vi "command-processor-old.vi"(8 "error in":errorcluster, 10 "Message Data Varient":variant, 11 "Queue in":refnum<queue>) -> (0 "error out":errorcluster, 1 "delta":dbl, 2 "executing command":string, 3 "output cluster":T1)   [LabVIEW 2017]
uses:
  Message Queue/Message Queue.lvlib
  Message Queue/Enqueue Message (Single).vi
  event-message-data.ctl
  Message Queue/Message Cluster.ctl
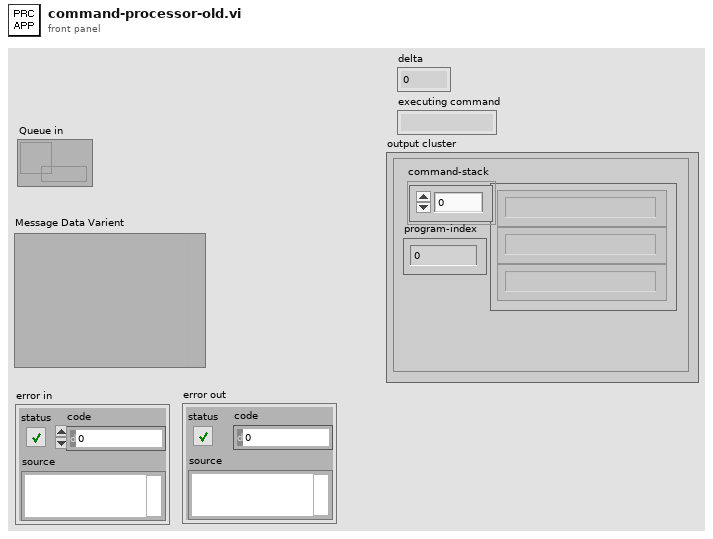
[diagram p1: front panel]
types:
  T1 = typedef "event-message-data.ctl" = cluster{"command-stack":string[], "program-index":i64}
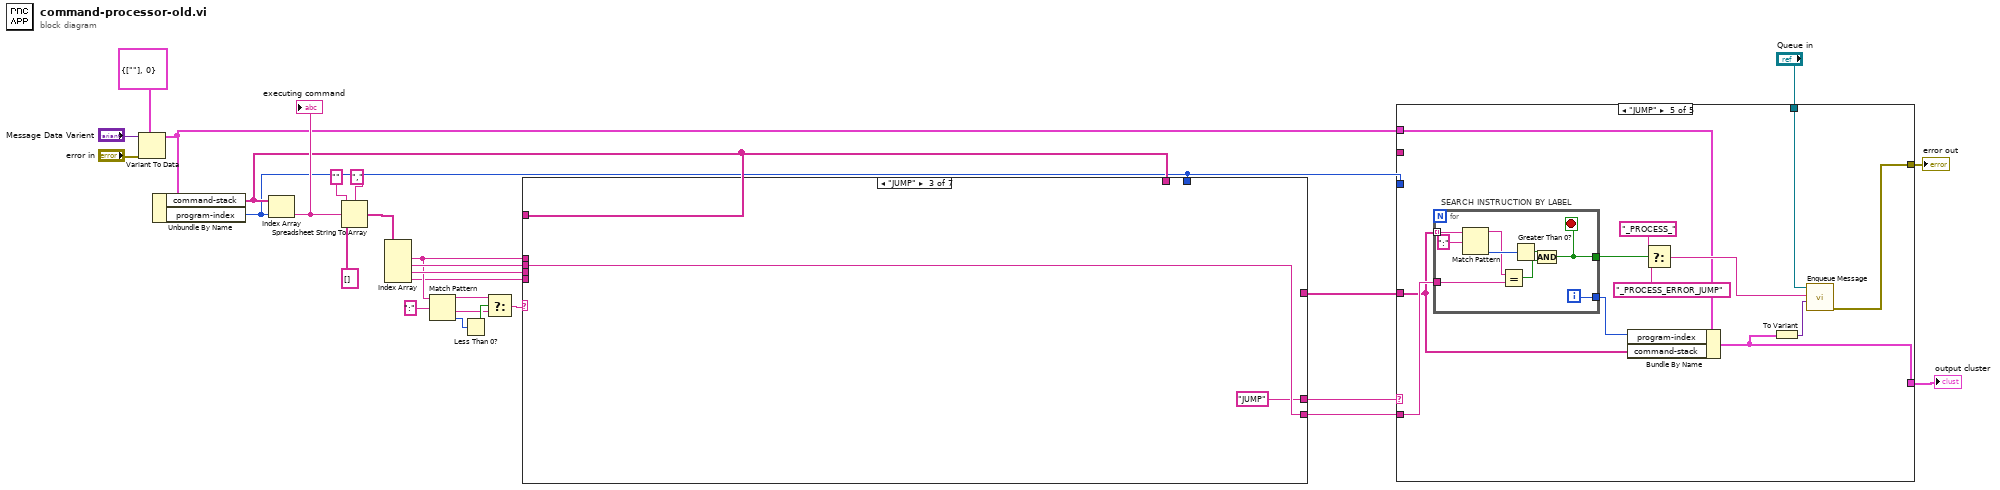
[diagram p0: block diagram]
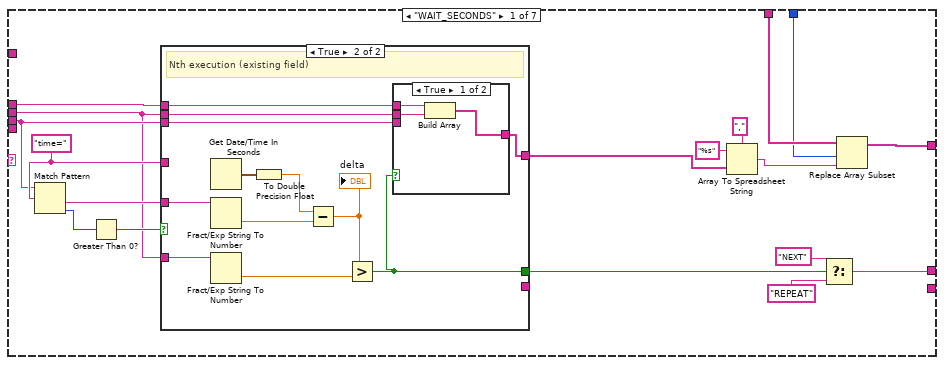
[diagram p2: hidden frame]
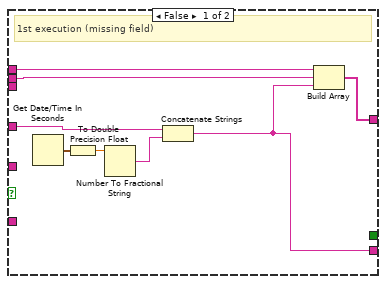
[diagram p3: hidden frame]
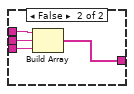
[diagram p4: hidden frame]
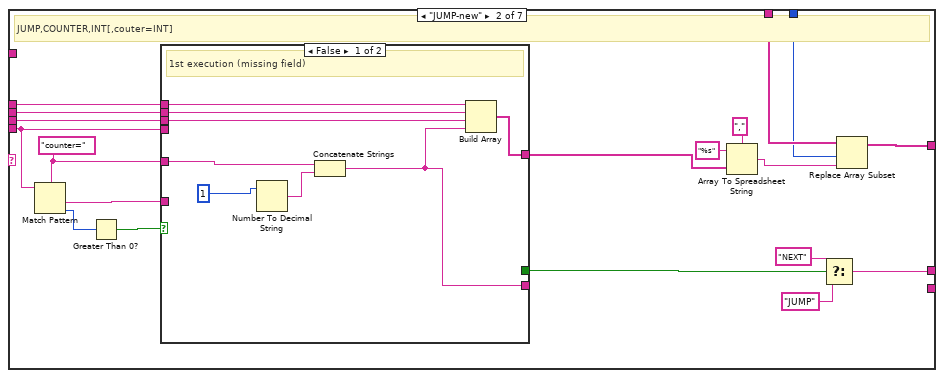
[diagram p5: hidden frame]
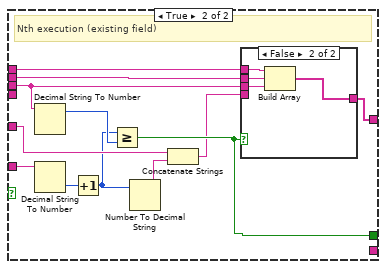
[diagram p6: hidden frame]
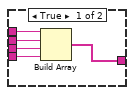
[diagram p7: hidden frame]
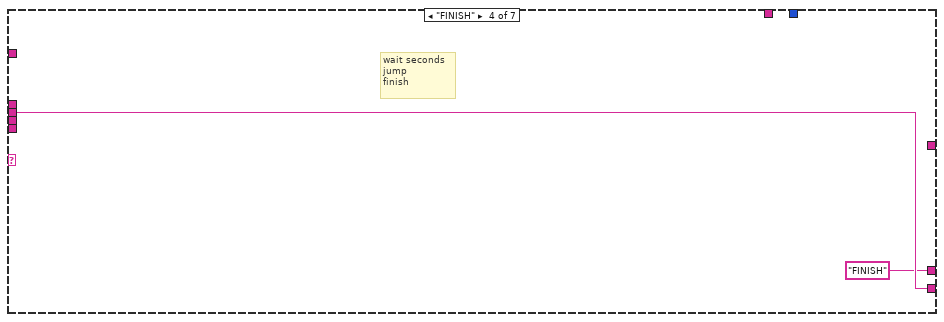
[diagram p8: hidden frame]
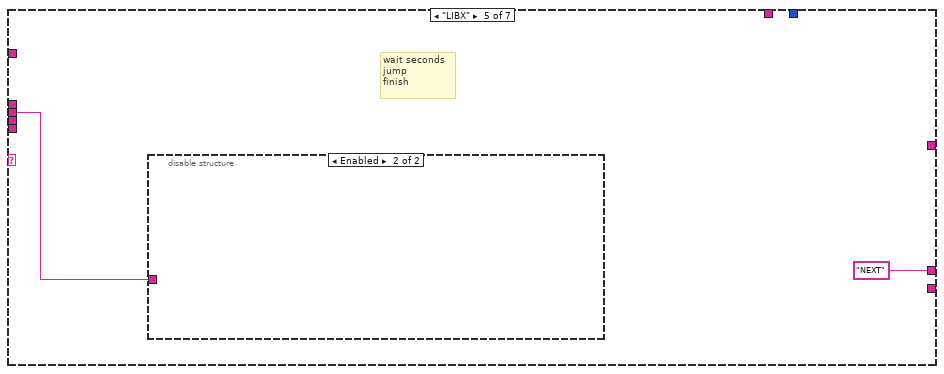
[diagram p9: hidden frame]
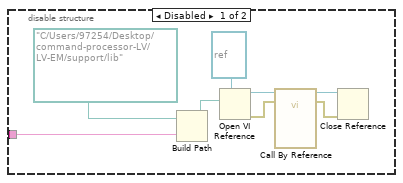
[diagram p10: hidden frame]
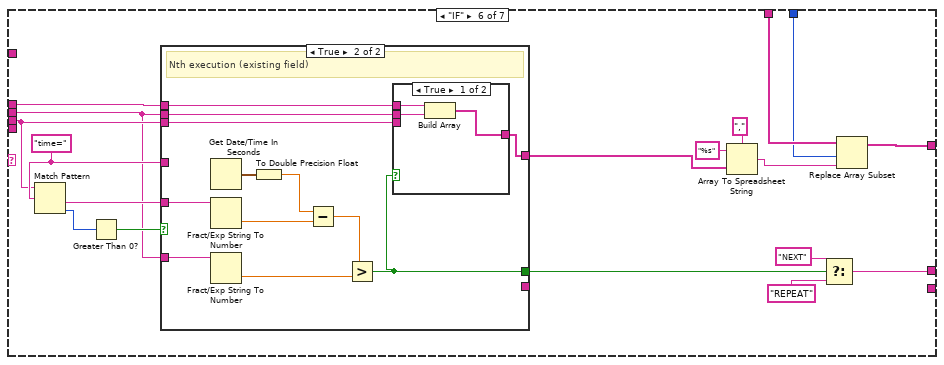
[diagram p11: hidden frame]
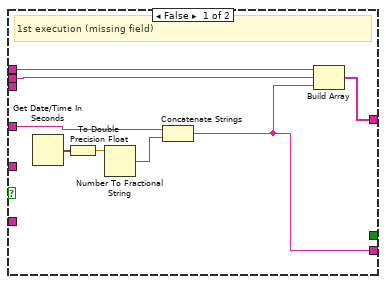
[diagram p12: hidden frame]
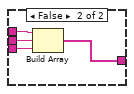
[diagram p13: hidden frame]
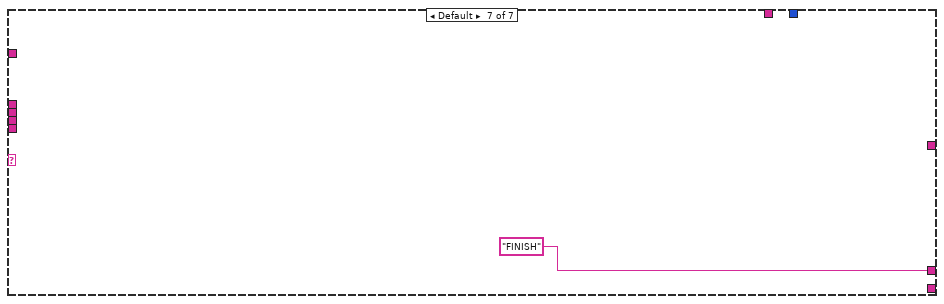
[diagram p14: hidden frame]
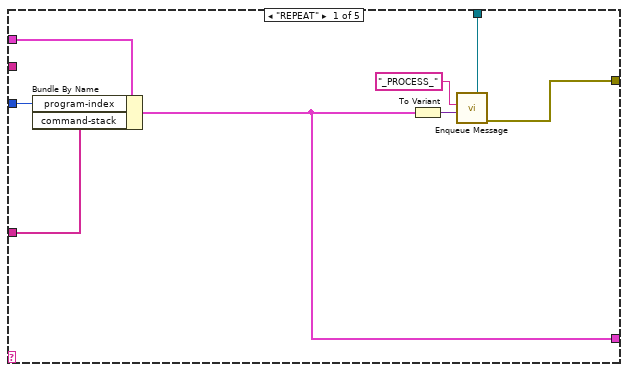
[diagram p15: hidden frame]
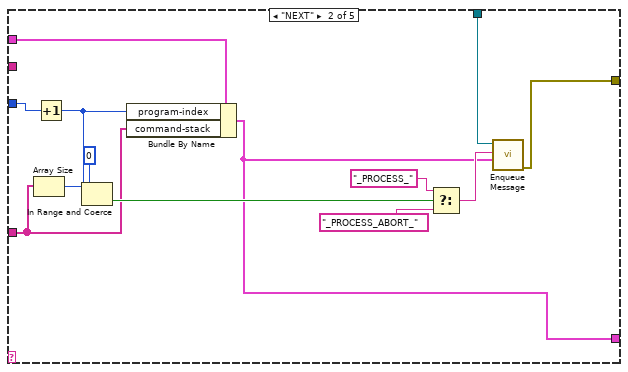
[diagram p16: hidden frame]
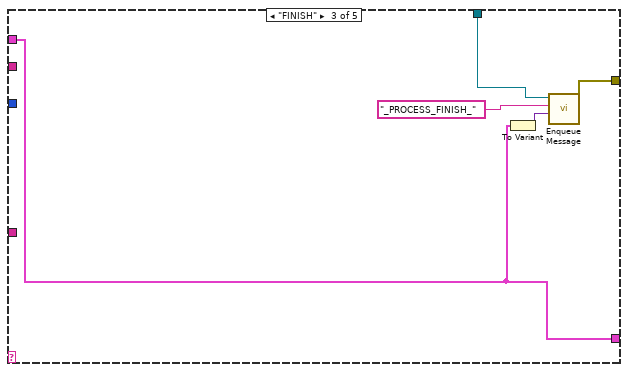
[diagram p17: hidden frame]
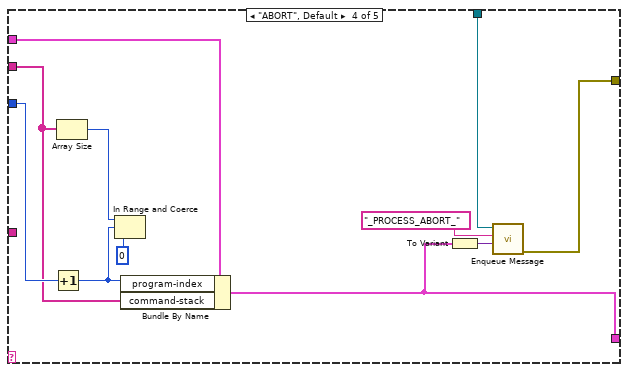
[diagram p18: hidden frame]
diagram:
  n1 = Variant To Data(error in="error in", type=T1 {"command-stack"=[""], "program-index"=0} ("process-unit"), Variant="Message Data Varient") -> (data=w5:T1)  [unwired: 1 out]
  n2 = Unbundle By Name(w5) -> ("command-stack"=w4:string[], "program-index"=w3:i64)
  n3 = Index Array(array=w4, index=w3) -> (element=w17:string)
  "executing command" <- w17
  n4 = Spreadsheet String To Array(delimiter (Tab)=",", format string="", spreadsheet string=w17, array type (2D Dbl)=string[] []) -> (array=w18:string[])
  n5 = Index Array(array=w18) -> (element #1=w6:string, element #2=w16:string, element #3=w15:string, element #4=w1:string)  [unwired: 4 in]
  n6 = Match Pattern(string=w6, regular expression=":") -> (before substring=w11:string, after substring=w10:string, offset past match=w13:i32)  [unwired: 1 in, 1 out]
  n7 = Less Than 0?(x=w13) -> (x < 0?=w12:bool)
  n8 = Select(t=w11, s=w12, f=w10) -> (s? t:f=w9:string)
  n9 = case shown="\"JUMP\"" w9 {
    tunnel: [w41 w87 "JUMP" ("format string") "FINISH" ("format string") "NEXT" ("format string") w148 "FINISH" ("format string")] -> w26
    tunnel: w16 -> [w33 w80 w122 w124 w125 w140 _]
    tunnel: w15 -> [w40 w86 _ _ _ w147 _]
    tunnel: [_ _ w122 w124 _ _ _] -> w8
    tunnel: w4 -> [_ _ _ _ _ _ _]
    tunnel: w6 -> [w34 w81 _ _ _ w141 _]
    tunnel: w4 -> [w31 w78 _ _ _ w138 _]
    tunnel: w3 -> [w29 w76 _ _ _ w136 _]
    tunnel: [w28 w75 _ _ _ w135 _] -> w2
    tunnel: w1 -> [_ w73 _ _ _ _ _]
    frame "WAIT_SECONDS" {
      w42 = "time=" ("regular expression")
      n10 = Match Pattern(string=w40, regular expression=w42) -> (after substring=w43:string, offset past match=w45:i32)  [unwired: 1 in, 2 out]
      n11 = Greater Than 0?(x=w45) -> (x > 0?=w44:bool)
      n12 = case shown="True" w44 {
        tunnel: [w47 _] -> _
        tunnel: w43 -> [_ w55]
        tunnel: w33 -> [_ w61]
        tunnel: w40 -> [_ w54]
        tunnel: w42 -> [w50 _]
        tunnel: [_ w59] -> w35
        tunnel: w34 -> [w49 w57]
        tunnel: w33 -> [w48 w56]
        tunnel: [w46 w58] -> w32
        frame False {
          # "1st execution (missing field)"
          n13 = Get Date/Time In Seconds() -> (seconds since 1Jan1904=w53:timestamp)
          n14 = To Double Precision Float(number=w53) -> (double precision float=w52:dbl)
          n15 = Number To Fractional String(number=w52) -> (F-format string=w51:string)  [unwired: 3 in]
          n16 = Concatenate Strings(w50, w51) -> (w47:string)
          n17 = Build Array(w49, w48, w47) -> (w46:string[])
        }
        frame True {
          # "Nth execution (existing field)"
          n18 = Get Date/Time In Seconds() -> (seconds since 1Jan1904=w65:timestamp)
          n19 = Fract/Exp String To Number(string=w55) -> (number=w63:dbl)  [unwired: 3 in, 1 out]
          n20 = Fract/Exp String To Number(string=w61) -> (number=w60:dbl)  [unwired: 3 in, 1 out]
          n21 = To Double Precision Float(number=w65) -> (double precision float=w64:dbl)
          n22 = Subtract(x=w64, y=w63) -> (x-y=w62:dbl)
          "delta" <- w62
          n23 = Greater?(x=w62, y=w60) -> (0:w59:bool)
          n24 = case shown="True" w59 {
            tunnel: [w68 w72] -> w58
            tunnel: w57 -> [w67 w70]
            tunnel: w56 -> [w66 w71]
            tunnel: w54 -> [_ w69]
            frame True {
              n25 = Build Array(w67, w66) -> (w68:string[])
            }
            frame False {
              n26 = Build Array(w70, w71, w69) -> (w72:string[])
            }
          }
        }
      }
      n27 = Array To Spreadsheet String(delimiter (Tab)=",", array=w32, 3:"%s" ("format string")) -> (spreadsheet string=w30:string)
      n28 = Select(t="NEXT" ("format string"), s=w35, f="REPEAT" ("format string")) -> (s? t:f=w41:string)
      n29 = Replace Array Subset(array=w31, new element=w30, index=w29) -> (w28:string[])
    }
    frame "JUMP-new" {
      w88 = "counter=" ("regular expression")
      # "JUMP,COUNTER,INT[,couter=INT]"
      n30 = Match Pattern(string=w73, regular expression=w88) -> (after substring=w89:string, offset past match=w91:i32)  [unwired: 1 in, 2 out]
      n31 = Greater Than 0?(x=w91) -> (x > 0?=w90:bool)
      n32 = case shown="False" w90 {
        tunnel: [w93 _] -> _
        tunnel: w89 -> [_ w108]
        tunnel: w86 -> [w92 w107]
        tunnel: w88 -> [w98 w103]
        tunnel: [_ w105] -> w82
        tunnel: w81 -> [w97 w110]
        tunnel: w80 -> [w96 w109]
        tunnel: [w95 w111] -> w79
        tunnel: w73 -> [_ _]
        frame False {
          # "1st execution (missing field)"
          n33 = Number To Decimal String(number=1) -> (decimal integer string=w99:string)  [unwired: 1 in]
          n34 = Concatenate Strings(w98, w99) -> (w93:string)
          n35 = Build Array(w97, w96, w92, w93) -> (w95:string[])
        }
        frame True {
          # "Nth execution (existing field)"
          n36 = Decimal String To Number(string=w107) -> (offset past number=w106:i32)  [unwired: 2 in, 1 out]
          n37 = Decimal String To Number(string=w108) -> (number=w102:i32)  [unwired: 2 in, 1 out]
          n38 = Increment(x=w102) -> (x+1=w100:i32)
          n39 = Greater Or Equal?(x=w100, y=w106) -> (x >= y?=w105:bool)
          n40 = Number To Decimal String(number=w100) -> (decimal integer string=w104:string)  [unwired: 1 in]
          n41 = Concatenate Strings(w103, w104) -> (w101:string)
          n42 = case shown="False" w105 {
            tunnel: [w116 w120] -> w111
            tunnel: w110 -> [w115 w118]
            tunnel: w109 -> [w114 w119]
            tunnel: w107 -> [w113 w117]
            tunnel: w101 -> [w112 _]
            frame True {
              n43 = Build Array(w115, w114, w113, w112) -> (w116:string[])
            }
            frame False {
              n44 = Build Array(w118, w119, w117) -> (w120:string[])
            }
          }
        }
      }
      n45 = Array To Spreadsheet String(delimiter (Tab)=",", array=w79, 3:"%s" ("format string")) -> (spreadsheet string=w77:string)
      n46 = Select(t="NEXT" ("format string"), s=w82, f="JUMP" ("format string")) -> (s? t:f=w87:string)
      n47 = Replace Array Subset(array=w78, new element=w77, index=w76) -> (w75:string[])
    }
    frame "JUMP" {
    }
    frame "FINISH" {
      # "wait seconds \njump\nfinish"
    }
    frame "LIBX" {
      # "wait seconds \njump\nfinish"
      n48 = disable-structure shown="Enabled" {
        disable-tunnel: w125 -> [w127 _]
        frame Disabled {
          n49 = Build Path(base path=path "C:/Users/97254/Desktop/command-processor-LV/LV-EM/support/lib" ("vi path"), name or relative path=w127) -> (appended path=w128:path)
          n50 = Open VI Reference(type specifier VI Refnum (for type only)=refnum<vi> refnum, vi path=w128) -> (vi reference=w132:refnum<vi>, error out=w129:errorcluster)  [unwired: 4 in]
          n51 = call-by-ref "?"(reference=w132, error in=w129) -> (reference out=w131:refnum<vi>, error out=w130:errorcluster)  [unwired: 12 in]
          n52 = Close Reference(reference=w131, error in (no error)=w130) -> ()  [unwired: 1 out]
        }
        frame Enabled {
        }
      }
    }
    frame "IF" {
      w149 = "time=" ("regular expression")
      n53 = Match Pattern(string=w147, regular expression=w149) -> (after substring=w150:string, offset past match=w152:i32)  [unwired: 1 in, 2 out]
      n54 = Greater Than 0?(x=w152) -> (x > 0?=w151:bool)
      n55 = case shown="True" w151 {
        tunnel: [w154 _] -> _
        tunnel: w150 -> [_ w162]
        tunnel: w140 -> [_ w168]
        tunnel: w147 -> [_ w161]
        tunnel: w149 -> [w157 _]
        tunnel: [_ w166] -> w142
        tunnel: w141 -> [w156 w164]
        tunnel: w140 -> [w155 w163]
        tunnel: [w153 w165] -> w139
        frame False {
          # "1st execution (missing field)"
          n56 = Get Date/Time In Seconds() -> (seconds since 1Jan1904=w160:timestamp)
          n57 = To Double Precision Float(number=w160) -> (double precision float=w159:dbl)
          n58 = Number To Fractional String(number=w159) -> (F-format string=w158:string)  [unwired: 3 in]
          n59 = Concatenate Strings(w157, w158) -> (w154:string)
          n60 = Build Array(w156, w155, w154) -> (w153:string[])
        }
        frame True {
          # "Nth execution (existing field)"
          n61 = Get Date/Time In Seconds() -> (seconds since 1Jan1904=w172:timestamp)
          n62 = Fract/Exp String To Number(string=w162) -> (number=w170:dbl)  [unwired: 3 in, 1 out]
          n63 = Fract/Exp String To Number(string=w168) -> (number=w167:dbl)  [unwired: 3 in, 1 out]
          n64 = To Double Precision Float(number=w172) -> (double precision float=w171:dbl)
          n65 = Subtract(x=w171, y=w170) -> (x-y=w169:dbl)
          n66 = Greater?(x=w169, y=w167) -> (0:w166:bool)
          n67 = case shown="True" w166 {
            tunnel: [w175 w179] -> w165
            tunnel: w164 -> [w174 w177]
            tunnel: w163 -> [w173 w178]
            tunnel: w161 -> [_ w176]
            frame True {
              n68 = Build Array(w174, w173) -> (w175:string[])
            }
            frame False {
              n69 = Build Array(w177, w178, w176) -> (w179:string[])
            }
          }
        }
      }
      n70 = Array To Spreadsheet String(delimiter (Tab)=",", array=w139, 3:"%s" ("format string")) -> (spreadsheet string=w137:string)
      n71 = Select(t="NEXT" ("format string"), s=w142, f="REPEAT" ("format string")) -> (s? t:f=w148:string)
      n72 = Replace Array Subset(array=w138, new element=w137, index=w136) -> (w135:string[])
    }
    frame Default {
    }
  }
  n73 = case shown="\"JUMP\"" w26 {
    tunnel: "Queue in" -> [w186 w198 w205 w211 w228]
    tunnel: [w185 w197 w204 w210 w227] -> w24
    tunnel: _ -> [_ _ _ w215 _]
    tunnel: w8 -> [_ _ _ _ w225]
    tunnel: w3 -> [w183 w201 _ w217 _]
    tunnel: [w182 w190 w202 w208 w226] -> w7
    tunnel: w5 -> [w184 w192 w202 w207 w219]
    tunnel: w2 -> [w181 w189 _ _ w218]
    frame "REPEAT" {
      n74 = Bundle By Name(cluster=w184, "program-index"=w183, "command-stack"=w181) -> (w182:T1)
      n75 = To Variant(anything=w182) -> (Variant=w187:variant)
      n76 = call-poly "Enqueue Message.vi"("Message Data"=w187, "Message"="_PROCESS_", "Message Queue"=w186) -> ("error out"=w185:errorcluster)  [unwired: 7 in, 1 out]
    }
    frame "NEXT" {
      n77 = Array Size(array=w189) -> (size(s)=w200:i32)
      n78 = Increment(x=w201) -> (x+1=w191:i64)
      n79 = In Range and Coerce(upper limit=w200, x=w191, lower limit=i64 0) -> (In Range?=w196:bool)  [unwired: 1 out]
      n80 = Bundle By Name(cluster=w192, "program-index"=w191, "command-stack"=w189) -> (w190:T1)
      n81 = Select(t="_PROCESS_" ("Message"), s=w196, f="_PROCESS_ABORT_" ("Message")) -> (s? t:f=w193:string)
      n82 = call-poly "Enqueue Message.vi"("Message Data"=w190, "Message"=w193, "Message Queue"=w198) -> ("error out"=w197:errorcluster)  [unwired: 7 in, 1 out]
    }
    frame "FINISH" {
      n83 = To Variant(anything=w202) -> (Variant=w206:variant)
      n84 = call-poly "Enqueue Message.vi"("Message Data"=w206, "Message"="_PROCESS_FINISH_", "Message Queue"=w205) -> ("error out"=w204:errorcluster)  [unwired: 7 in, 1 out]
    }
    frame "ABORT", Default {
      n85 = Increment(x=w217) -> (x+1=w216:i64)
      n86 = Array Size(array=w215) -> (size(s)=w214:i32)
      n87 = In Range and Coerce(upper limit=w214, x=w216, lower limit=i64 0) -> ()  [unwired: 2 out]
      n88 = Bundle By Name(cluster=w207, "program-index"=w216, "command-stack"=w215) -> (w208:T1)
      n89 = To Variant(anything=w208) -> (Variant=w212:variant)
      n90 = call-poly "Enqueue Message.vi"("Message Data"=w212, "Message"="_PROCESS_ABORT_", "Message Queue"=w211) -> ("error out"=w210:errorcluster)  [unwired: 7 in, 1 out]
    }
    frame "JUMP" {
      n91 = for "SEARCH INSTRUCTION BY LABEL" {
        tunnel: w218 -> [w236] mode=indexing
        tunnel: [w235] -> w224
        tunnel: w225 -> [w233]
        tunnel: [w230] -> w222
        i -> [w235]
        stop <- w230 stop-if-true
        n92 = Match Pattern(string=w236, regular expression=":") -> (before substring=w232:string, offset past match=w237:i32)  [unwired: 1 in, 2 out]
        n93 = Equal?(x=w232, y=w233) -> (x = y?=w231:bool)
        n94 = Greater Than 0?(x=w237) -> (x > 0?=w234:bool)
        n95 = Compound Arithmetic op=AND(w234, w231) -> (w230:bool)
      }
      n96 = Bundle By Name(cluster=w219, "program-index"=w224, "command-stack"=w218) -> (w226:T1)
      n97 = Select(t="_PROCESS_" ("Message"), s=w222, f="_PROCESS_ERROR_JUMP" ("Message")) -> (s? t:f=w220:string)
      n98 = To Variant(anything=w226) -> (Variant=w229:variant)
      n99 = call-poly "Enqueue Message.vi"("Message Data"=w229, "Message"=w220, "Message Queue"=w228) -> ("error out"=w227:errorcluster)  [unwired: 7 in, 1 out]
    }
  }
  "error out" <- w24
  "output cluster" <- w7
